vi "TIO Data Stream Column Names.vi"(1 "Raw Data":T1={"stream ID"=0, "Sample Number"=417475, "Raw Data"=":-É%a\u0000J1\n\u0000É†Eï>tn\u0013Áõ9FÀó\u0010Ÿ<wm\u0010<u;Î;"}, 2 "TIO State":T2={"Awaiting REP"=FALSE, "REQ ID"=500, "streams in"=[], "sources"=[], "timebases"=[]}) -> (0 "String":string)   [LabVIEW 2017]
panel:
  # "TIO Data Column Names"
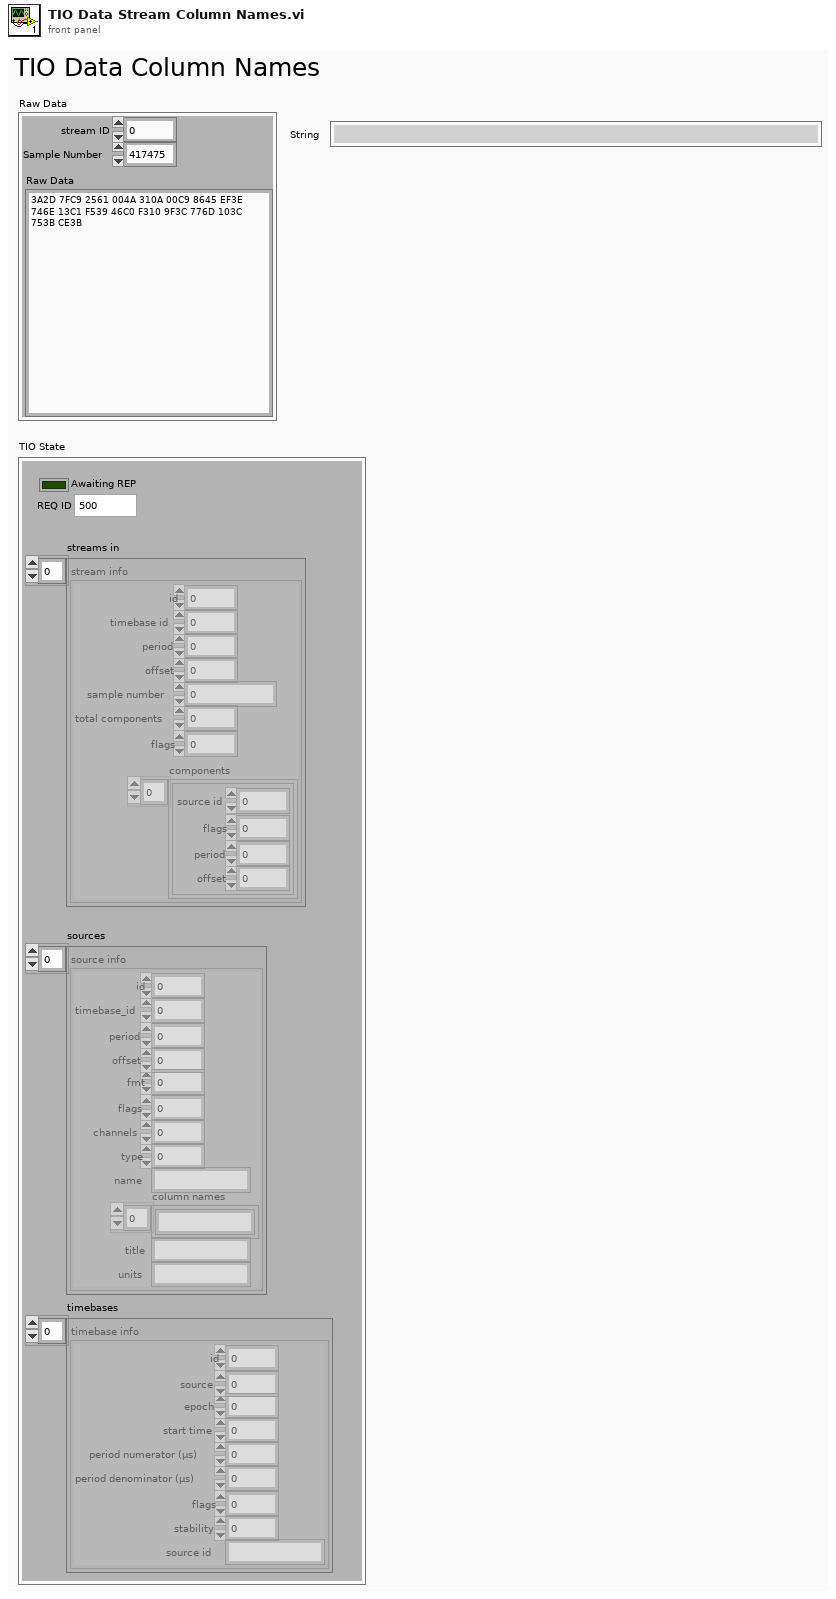
[diagram p1: front panel]
types:
  T1 = cluster{"stream ID":u16, "Sample Number":u32, "Raw Data":string}
  T2 = cluster{"Awaiting REP":bool, "REQ ID":u32, "streams in":cluster{"id":u16, "timebase id":u16, "period":u32, "offset":u32, "sample number":u64, "total components":u16, "flags":u16, "components":cluster{"source id":u16, "flags":u16, "period":u32, "offset":u32}[]}[], "sources":cluster{"id":u16, "timebase_id":u16, "period":u32, "offset":u32, "fmt":i32, "flags":u16, "channels":u16, "type":u8, "name":string, "column names":string[], "title":string, "units":string}[], "timebases":cluster{"id":u16, "source":u16, "epoch":u32, "start time":u32, "period numerator (µs)":i32, "period denominator (µs)":u16, "flags":u16, "stability":u8, "source id":string}[]}
  T3 = cluster{"id":u16, "timebase_id":u16, "period":u32, "offset":u32, "fmt":i32, "flags":u16, "channels":u16, "type":u8, "name":string, "column names":string[], "title":string, "units":string}[]
  T4 = cluster{"id":u16, "timebase id":u16, "period":u32, "offset":u32, "sample number":u64, "total components":u16, "flags":u16, "components":cluster{"source id":u16, "flags":u16, "period":u32, "offset":u32}[]}[]
  T5 = cluster{"id":u16, "timebase id":u16, "period":u32, "offset":u32, "sample number":u64, "total components":u16, "flags":u16, "components":cluster{"source id":u16, "flags":u16, "period":u32, "offset":u32}[]}
  T6 = cluster{"source id":u16, "flags":u16, "period":u32, "offset":u32}[]
  T7 = cluster{"id":u16, "timebase_id":u16, "period":u32, "offset":u32, "fmt":i32, "flags":u16, "channels":u16, "type":u8, "name":string, "column names":string[], "title":string, "units":string}
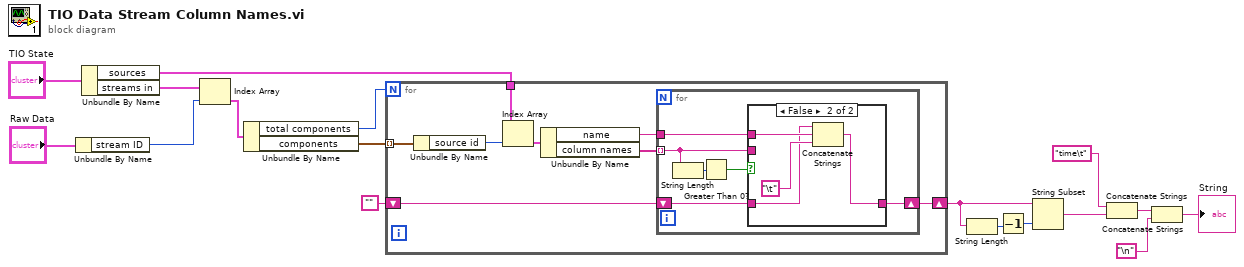
[diagram p0: block diagram]
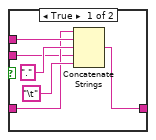
[diagram p2: hidden frame]
diagram:
  n1 = Unbundle By Name("Raw Data") -> ("stream ID"=w15:u16)
  n2 = Unbundle By Name("TIO State") -> ("sources"=w10:T3, "streams in"=w14:T4)
  n3 = Index Array(array=w14, index=w15) -> (element=w13:T5)
  n4 = Unbundle By Name(w13) -> ("total components"=w12:u16, "components"=w11:T6)
  n5 = for {
    N: w12 -> [_]
    tunnel: w11 -> [w25] mode=indexing
    tunnel: w10 -> [w24]
    shift-right: [w18] -> w6
    shift-left: "" -> [w19]
    n6 = Unbundle By Name(w25) -> ("source id"=w23:u16)
    n7 = Index Array(array=w24, index=w23) -> (element=w22:T7)
    n8 = Unbundle By Name(w22) -> ("name"=w20:string, "column names"=w21:string[])
    n9 = for {
      tunnel: w21 -> [w28] mode=indexing
      tunnel: w20 -> [w31]
      shift-right: [w26] -> w18
      shift-left: w19 -> [w30]
      n10 = String Length(string=w28) -> (length=w29:i32)
      n11 = Greater Than 0?(x=w29) -> (x > 0?=w27:bool)
      n12 = case shown="False" w27 {
        tunnel: w31 -> [w36 w41]
        tunnel: [w34 w39] -> w26
        tunnel: w30 -> [w33 w38]
        tunnel: w28 -> [w32 _]
        frame True {
          n13 = Concatenate Strings(w33, w36, ".", w32, "\t") -> (w34:string)
        }
        frame False {
          n14 = Concatenate Strings(w38, w41, "\t") -> (w39:string)
        }
      }
    }
  }
  n15 = String Length(string=w6) -> (length=w7:i32)
  n16 = Decrement(x=w7) -> (x-1=w8:i32)
  n17 = String Subset(string=w6, length (rest)=w8) -> (substring=w3:string)  [unwired: 1 in]
  n18 = Concatenate Strings("time\t", w3) -> (w2:string)
  n19 = Concatenate Strings(w2, "\n") -> (→"String":string)
